vi "Test - Add Property to Schema.vi"   [LabVIEW 2020, in "JSON Schema Generator.lvlib"]
uses:
  JSON Schema Generator.lvlib
  <vilib>/addons/_JKI Toolkits/Caraya/classes/Test/Test.lvclass
  <vilib>/addons/_JKI Toolkits/Caraya/classes/Assert/Assert.lvclass
  <vilib>/JDP Science/JSONtext/JSONtext.lvlib
  <vilib>/addons/_JKI Toolkits/Caraya/classes/Assert/Assert Equal Value_Variant.vi
  <vilib>/addons/_JKI Toolkits/Caraya/classes/Assert/Assert Not Error.vi
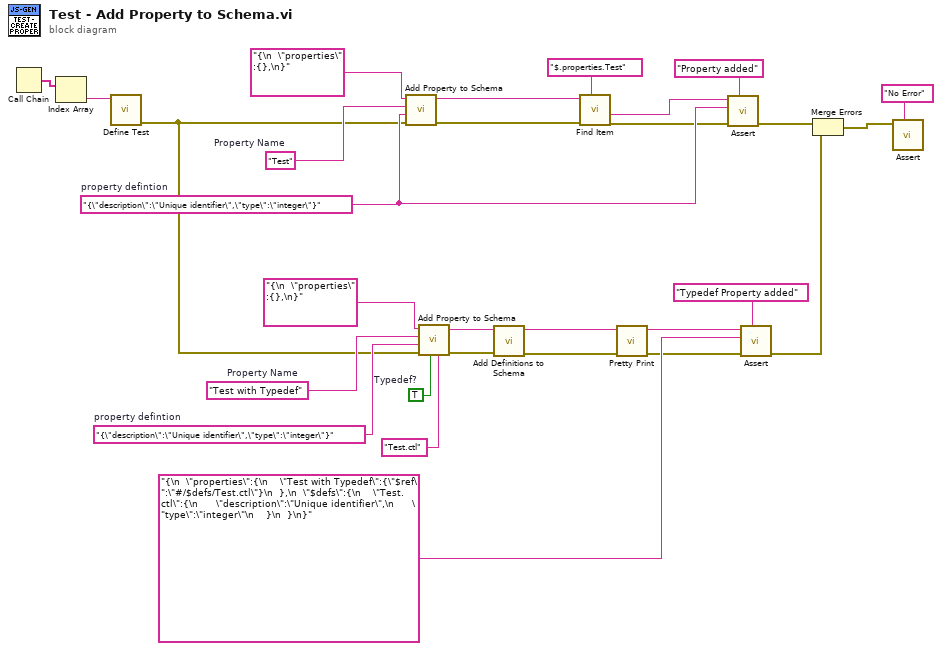
[diagram p0: block diagram]
diagram:
  w9 = TRUE  # Typedef?
  w14 = "{\"description\":\"Unique identifier\",\"type\":\"integer\"}"  # property defintion
  w16 = "Test with Typedef"  # Property Name
  w20 = "{\"description\":\"Unique identifier\",\"type\":\"integer\"}"  # property defintion
  w23 = "Test"  # Property Name
  n1 = Call Chain() -> (call chain=w29:string[])
  n2 = Index Array(array=w29) -> (element=w28:string)  [unwired: 1 in]
  n3 = call <vilib>:"Define Test.vi"("Label (VI Title)"=w28) -> ("error out"=w13:errorcluster)  [unwired: 9 in, 1 out]
  n4 = call "Add Property to Schema.vi"("error in"=w13, "JSON Schema Property in"=w20, "Property Name"=w23, "JSON Schema in"="{\n  \"properties\" :{},\n}") -> ("error out"=w7:errorcluster, "JSON Schema out"=w8:string)  [unwired: 6 in]
  n5 = call "Add Property to Schema.vi"("Typedef Name"="Test.ctl", "Typedef?"=w9, "error in"=w13, "JSON Schema Property in"=w14, "Property Name"=w16, "JSON Schema in"="{\n  \"properties\" :{},\n}") -> ("error out"=w5:errorcluster, "JSON Schema out"=w6:string)  [unwired: 4 in]
  n6 = call "Add Definitions to Schema.vi"("error in (no error)"=w5, "JSON In"=w6) -> ("error out"=w2:errorcluster, "JSON Out"=w4:string)  [unwired: 8 in]
  n7 = call <vilib>:"Find Item.vi"("$Path or Item Name"="$.properties.Test", "error in (no error)"=w7, "JSON"=w8) -> ("error out"=w19:errorcluster, "<JSON>"=w21:string)  [unwired: 5 in, 2 out]
  n8 = call <vilib>:"Pretty Print.vi"("error in (no error)"=w2, "JSON"=w4) -> ("error out"=w1:errorcluster, "<JSON>"=w3:string)  [unwired: 7 in, 1 out]
  n9 = call-poly <vilib>:"Assert.vi"("Label"="Property added", "error in (no error)"=w19, "Actual"=w20, "Expected"=w21) -> ("error out"=w26:errorcluster)  [unwired: 6 in, 1 out]
  n10 = call-poly <vilib>:"Assert.vi"("Label"="Typedef Property added", "error in (no error)"=w1, "Actual"="{\n  \"properties\":{\n    \"Test with Typedef\":{\"$ref\":\"#/$defs/Test.ctl\"}\n  },\n  \"$defs\":{\n    \"Test.ctl\":{\n      \"description\":\"Unique identifier\",\n      \"type\":\"integer\"\n    }\n  }\n}", "Expected"=w3) -> ("error out"=w11:errorcluster)  [unwired: 6 in, 1 out]
  n11 = Merge Errors(w26, w11) -> (w24:errorcluster)
  n12 = call-poly <vilib>:"Assert.vi"("Label"="No Error", "Not Error?"=w24) -> ()  [unwired: 8 in, 2 out]
